vi "Set Not Implemented Error.vi"(7 "VI Reference":refnum<vi>, 8 "error in (no error)":errorcluster, 11 "BS120x in":refnum<class "BS120x.lvclass">) -> (0 "error out":errorcluster, 3 "BS120x out":refnum<class "BS120x.lvclass">)   [LabVIEW 2021, in "BS120x Driver.lvlib" / "BS120x.lvclass"]
uses:
  BS120x.lvclass
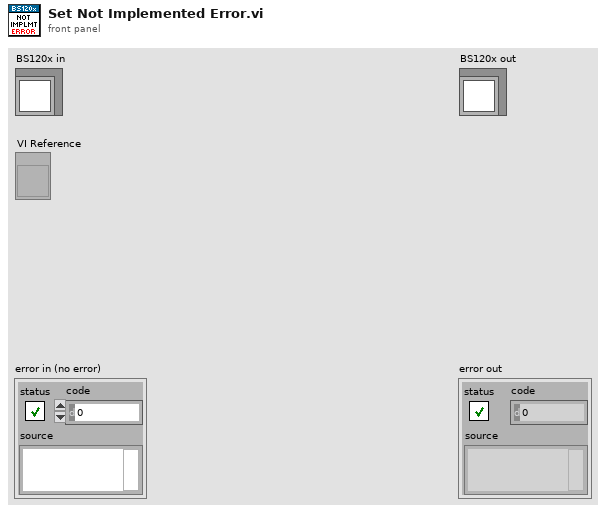
[diagram p1: front panel]
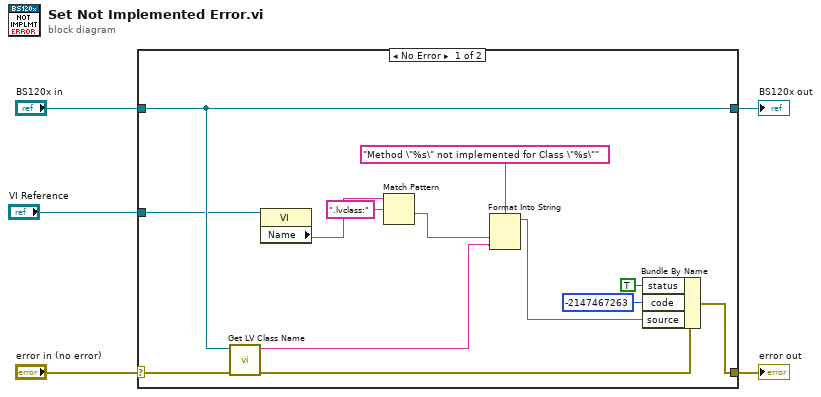
[diagram p0: block diagram]
diagram:
  n1 = case shown="No Error" "error in (no error)" {
    selector: "error in (no error)" -> [w17 w20]
    tunnel: [w9 w20] -> w4
    tunnel: [w18 w19] -> w2
    tunnel: "BS120x in" -> [w18 w19]
    tunnel: "VI Reference" -> [w13 _]
    frame No Error {
      n2 = call <vilib>:"Get LV Class Name.vi"("error in (no error)"=w17, "object"=w18) -> ("error out"=w16:errorcluster, "class name"=w11:string)  [unwired: 8 in]
      n3 = property class="VI"(reference=w13) -> ("Name"=w7:string)  [unwired: 1 in, 2 out]
      n4 = Match Pattern(string=w7, regular expression=".lvclass:") -> (after substring=w6:string)  [unwired: 1 in, 3 out]
      n5 = Format Into String(format string="Method \"%s\" not implemented for Class \"%s\"", w6, w11) -> (resulting string=w10:string)  [unwired: 2 in, 1 out]
      n6 = Bundle By Name(cluster=w16, "status"=TRUE, "code"=-2147467263, "source"=w10) -> (w9:errorcluster)
    }
    frame Error {
    }
  }
  "error out" <- w4
  "BS120x out" <- w2
